vi "DB Tools Get Types.vi"(4 "error in (no error)":errorcluster, 6 "file?":bool, 7 "connection reference":T2) -> (0 "error out":errorcluster, 1 "database":T1, 2 "data types":string[](array[string]), 3 "connection reference out":T2)   [LabVIEW 2012, in "NI_Database_API_64.lvlib"]
doc: "Returns the data types and database supported by the specified connection reference. If the file? input is TRUE, the VI uses a user-supplied file to determine the native database types."
uses:
  NI_Database_API_64.lvlib
  Connection.llb/Conn ObjectReference.ctl
  DB Tools Database.ctl
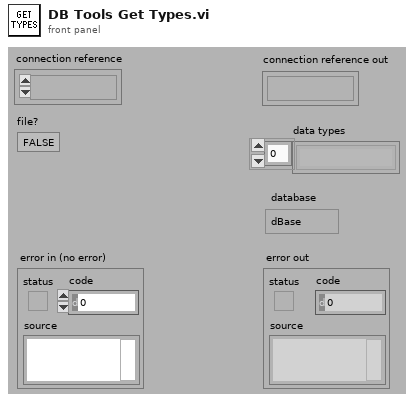
[diagram p1: front panel]
types:
  T1 = typedef "NI_Database_API_64.lvlib/DB Tools Database.ctl" = enum16{"dBase", "Jet", "SQL Server", "Oracle"}
  T2 = typedef "NI_Database_API_64.lvlib/Conn ObjectReference.ctl" = refnum<k1>
  T3 = typedef "NI_Database_API_64.lvlib/Conn DataMembers.ctl" = cluster{"ADODB._Connection":refnum<k7>, "recordset objects":i32, "command objects":i32}
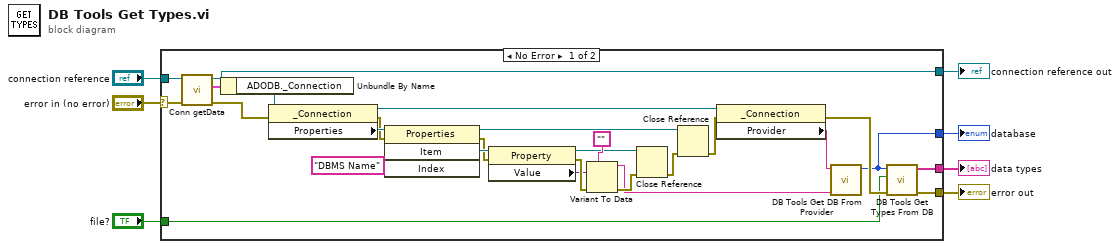
[diagram p0: block diagram]
diagram:
  n1 = case shown="No Error" "error in (no error)" {
    selector: "error in (no error)" -> [w8 w36]
    tunnel: [w29 w36] -> w7
    tunnel: [w16 _] -> w6
    tunnel: [w15 _] -> w5
    tunnel: "file?" -> [w14 _]
    tunnel: "connection reference" -> [w12 w35]
    tunnel: [w9 w35] -> w2
    frame No Error {
      n2 = call "Conn getData.vi"("error in (no error)"=w8, "connection reference"=w12) -> ("error out"=w11:errorcluster, "data"=w13:T3, "connection reference out"=w9:T2)  [unwired: 2 in, 1 out]
      n3 = Unbundle By Name(w13) -> ("ADODB._Connection"=w10:refnum<k7>)
      n4 = property class="_Connection"(reference=w10, error in=w11) -> (reference out=w20:refnum<k7>, error out=w27:errorcluster, "Properties"=w28:refnum<k7>)
      n5 = invoke class="Properties" method="Item"(reference=w28, error in=w27, "Index"="DBMS Name") -> (reference out=w26:refnum<k7>, error out=w24:errorcluster, "Item"=w25:refnum<k7>)  [unwired: 1 in, 1 out]
      n6 = property class="Property"(reference=w25, error in=w24) -> (reference out=w23:refnum<k7>, error out=w22:errorcluster, "Value"=w21:variant)
      n7 = Variant To Data(error in=w22, type="", Variant=w21) -> (data=w30:string, error out=w32:errorcluster)
      n8 = Close Reference(reference=w23, error in (no error)=w32) -> (error out=w31:errorcluster)
      n9 = Close Reference(reference=w26, error in (no error)=w31) -> (error out=w19:errorcluster)
      n10 = property class="_Connection"(reference=w20, error in=w19) -> (error out=w17:errorcluster, "Provider"=w18:string)  [unwired: 1 out]
      n11 = call "DB Tools Get DB From Provider.vi"("DBMS Name"=w30, "Provider"=w18) -> ("database"=w16:T1)  [unwired: 5 in]
      n12 = call "DB Tools Get Types From DB.vi"("error in (no error)"=w17, "file?"=w14, "database"=w16) -> ("error out"=w29:errorcluster, "data types"=w15:string[])  [unwired: 3 in]
    }
    frame Error {
    }
  }
  "connection reference out" <- w2
  "error out" <- w7
  "database" <- w6
  "data types" <- w5
